vi "Periodic Tasks.vi"(8 "error in":errorcluster) -> ()   [LabVIEW 2020]
doc: "This VI runs in parallel to other tasks. It can contain as many user-defined periodic loops as you need. These can carry out PID or other sorts of timed response."
uses:
  <vilib>/Rock Robotics/WPI/Solenoid/WPI_SolenoidValue.ctl
  <vilib>/Rock Robotics/WPI/ThirdParty/Phoenix-LabVIEW/Motor Controller/Controls/CTRE_Phoenix_MotorControl_ControlMode.ctl
  <vilib>/Rock Robotics/WPI/Utilities/WPI_GetSetVariantRefNum.vi
  Robot Global Data.vi
  <vilib>/Rock Robotics/WPI/Solenoid/WPI_SolenoidSetEnum.vi
  <vilib>/Rock Robotics/Network Tables/NT Write Numeric Array.vi
  <vilib>/Analysis/Matrix/NI_Matrix.lvlib
  <vilib>/Rock Robotics/Network Tables/NT Read Boolean.vi
  <vilib>/Rock Robotics/Network Tables/NT Read String.vi
  <vilib>/Analysis/Matrix/Numeric/Conversions/Matrix To Array - RM.vi
  <vilib>/Utility/file.llb/Write Delimited Spreadsheet (DBL).vi
panel:
  in  "Co Axes Cluster":T1
  in  "Co Button Cluster":T2
  in  "Driver Axes Cluster":T3
  in  "Driver Button Cluster":T4
  out "ArmExtensionEncoderData":i32
  out "ArmPivotEncoderData":i32
  in  "ArmPneumaticControl":T5
  in  "ArmPivotControl":dbl
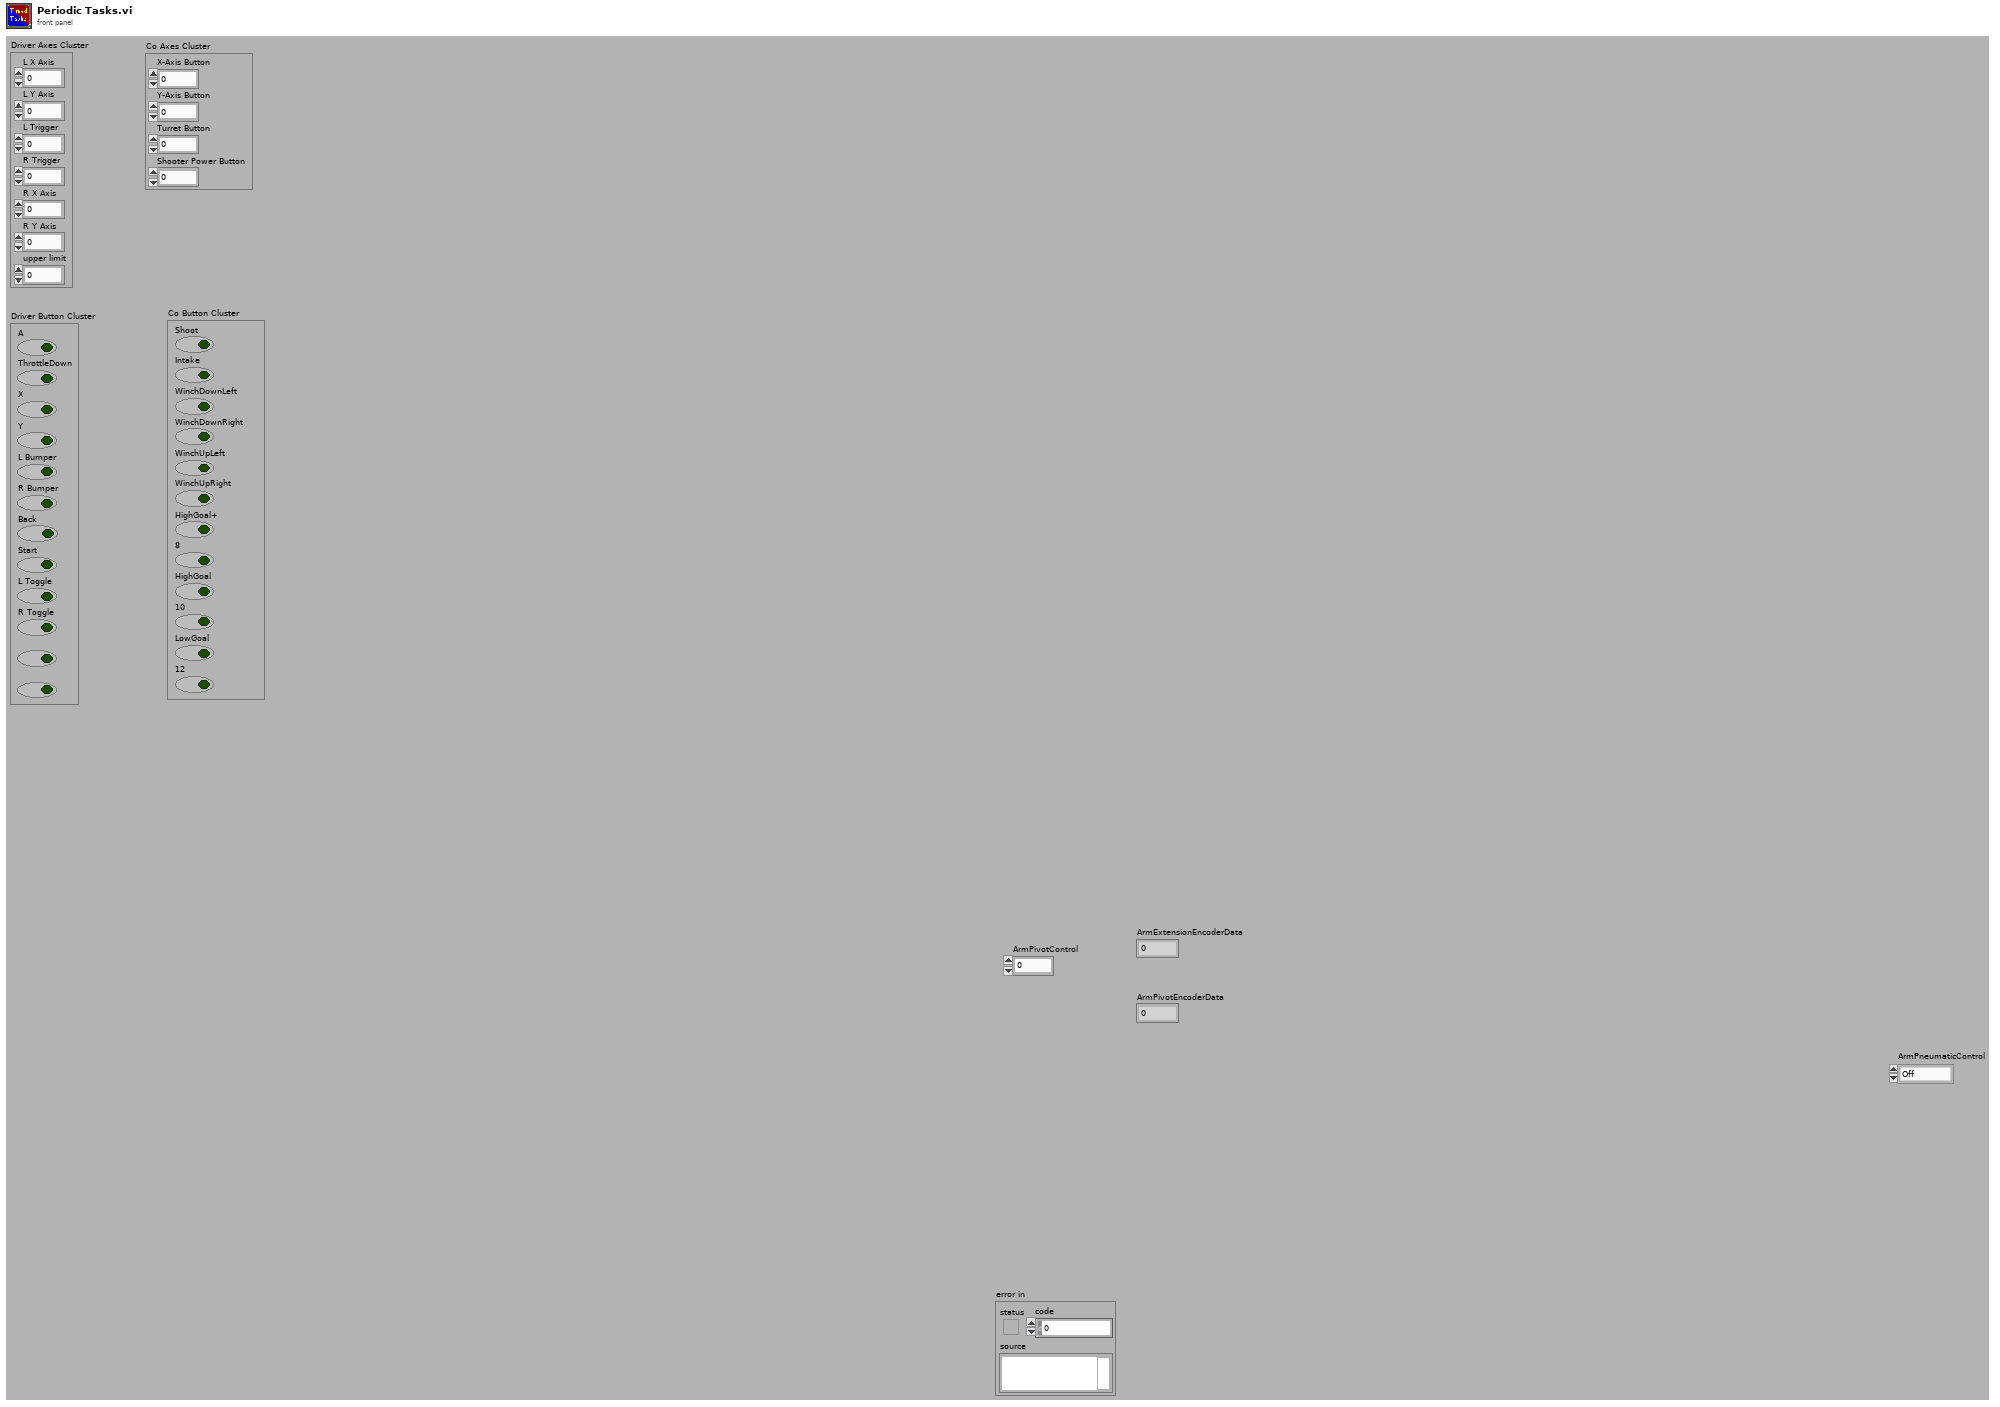
[diagram p1: front panel]
types:
  T1 = cluster{"X-Axis Button":dbl, "Y-Axis Button":dbl, "Turret Button":dbl, "Shooter Power Button":dbl}
  T2 = cluster{"Shoot":bool, "Intake":bool, "WinchDownLeft":bool, "WinchDownRight":bool, "WinchUpLeft":bool, "WinchUpRight":bool, "HighGoal+":bool, "8":bool, "HighGoal":bool, "10":bool, "LowGoal":bool, "12":bool}
  T3 = cluster{"L X Axis":dbl, "L Y Axis":dbl, "L Trigger":dbl, "R Trigger":dbl, "R X Axis":dbl, "R Y Axis":dbl, "upper limit":dbl}
  T4 = cluster{"A":bool, "ThrottleDown":bool, "X":bool, "Y":bool, "L Bumper":bool, "R Bumper":bool, "Back\n":bool, "Start":bool, "L Toggle":bool, "R Toggle":bool, bool, bool}
  T5 = typedef "WPI_SolenoidValue.ctl" = enum16{"Off", "On", "Forward", "Reverse"}
  T6 = typedef "WPI_RobotDriveDevRef.ctl" = cluster{"DevStatus":errorcluster, "Motors[]":T7[], "Square Inputs":bool, "Max Output":dbl}
  T7 = typedef "WPI_MotorControlDeviceRef.ctl" = cluster{"DeviceStatus":errorcluster, "Type":T8, "PWM":cluster{"PWM Channel":T9, "DeadBand":T10}, "CAN":cluster{"Device Number":u8, "SetOutput VI Ref":variant, "GetOutput VI Ref":variant, "Enable VI Ref":variant, "Disable VI Ref":variant, "Data":variant}, "Invert":bool, "DIO PWM":cluster{"PWM \"Enable\" Channel":T9, "DIOChannel":T11, "PWM Rate":dbl}}
  T8 = typedef "WPI_MotorControlType.ctl" = enum16{"PWM", "CAN", "DIO PWM"}
  T9 = typedef "FPGA_DIOPWMChannel.ctl" = enum8{"PWM 0", "PWM 1", "PWM 2", "PWM 3", "PWM 4", "PWM 5", "PWM 6", "PWM 7", "PWM 8", "PWM 9", "PWM MXP 0", "PWM MXP 1", "PWM MXP 2", "PWM MXP 3", "PWM MXP 4", "PWM MXP 5", "PWM MXP 6", "PWM MXP 7", "PWM MXP 8", "PWM MXP 9", "Invalid"}
  T10 = typedef "WPI_PWMDeadband.ctl" = cluster{"Name":string, "maxPositivePwm":i32, "minPositivePwm":i32, "centerPwm":i32, "maxNegativePwm":i32, "minNegativePwm":i32, "angularRange":u16}
  T11 = typedef "FPGA_DIOChannel.ctl" = enum8{"DIO 0", "DIO 1", "DIO 2", "DIO 3", "DIO 4", "DIO 5", "DIO 6", "DIO 7", "DIO 8", "DIO 9", "DIO MXP 0", "DIO MXP 1", "DIO MXP 2", "DIO MXP 3", "DIO MXP 4", "DIO MXP 5", "DIO MXP 6", "DIO MXP 7", "DIO MXP 8", "DIO MXP 9", "DIO MXP 10", "DIO MXP 11", "DIO MXP 12", "DIO MXP 13", "DIO MXP 14", "DIO MXP 15", "SPI Port CS1", "SPI Port CS2", "SPI Port CS3", "SPI Port MISO", "SPI Port MOSI", "Invalid"}
  T12 = typedef "WPI_JoystickDevRef.ctl" = cluster{"Device":T13}
  T13 = typedef "WPI_JoystickDeviceEnum.ctl" = enum16{"USB 0", "USB 1", "USB 2", "USB 3", "USB 4", "USB 5"}
  T14 = typedef "CTRE_Phoenix_MotorControl_ControlMode.ctl" = u16
  T15 = cluster{"JoystickDevRef":T12, "JoystickDevRef":T12, "RobotDriveDevRef":T6}
  T16 = typedef "WPI_DriverStationRobotMode2.ctl" = enum16{"Autonomous Disabled", "Autonomous Enabled", "Teleop Disabled", "Teleop Enabled", "Disconnected", "Finish", "Test Disabled", "Test Enabled", "Emergency Stopped"}
  T17 = typedef "WPI_SolenoidDevRef.ctl" = cluster{"DevStatus":errorcluster, "Pneumatics Control Module":u8, "Forward Solenoid Channel":T18, "Reverse Solenoid Channel":T18}
  T18 = typedef "WPI_SolenoidChannel.ctl" = enum8{"Solenoid 0", "Solenoid 1", "Solenoid 2", "Solenoid 3", "Solenoid 4", "Solenoid 5", "Solenoid 6", "Solenoid 7", "Solenoid 8", "Solenoid 9", "Solenoid 10", "Solenoid 11", "Solenoid 12", "Solenoid 13", "Solenoid 14", "Solenoid 15", "Invalid"}
  T19 = typedef "WPI_DigitalInputDevRef.ctl" = cluster{"DevStatus":errorcluster, "DIO Channel":T11}
  T20 = typedef "WPI_AnalogChannelDevRef.ctl" = cluster{"DevStatus":errorcluster, "Analog Channel":T21}
  T21 = typedef "FPGA_AIChannel.ctl" = enum8{"AI 0", "AI 1", "AI 2", "AI 3", "AI MXP 0", "AI MXP 1", "AI MXP 2", "AI MXP 3", "Invalid"}
  T22 = typedef "CTRE_CANifier_DeviceRef.ctl" = cluster{"DeviceStatus":errorcluster, "Device Number":u8, "Handle":u64, "UsageFrame":u32, "Library Path":path}
  T23 = typedef "NI_Matrix.lvlib/RealMatrix.ctl" = dbl[][]
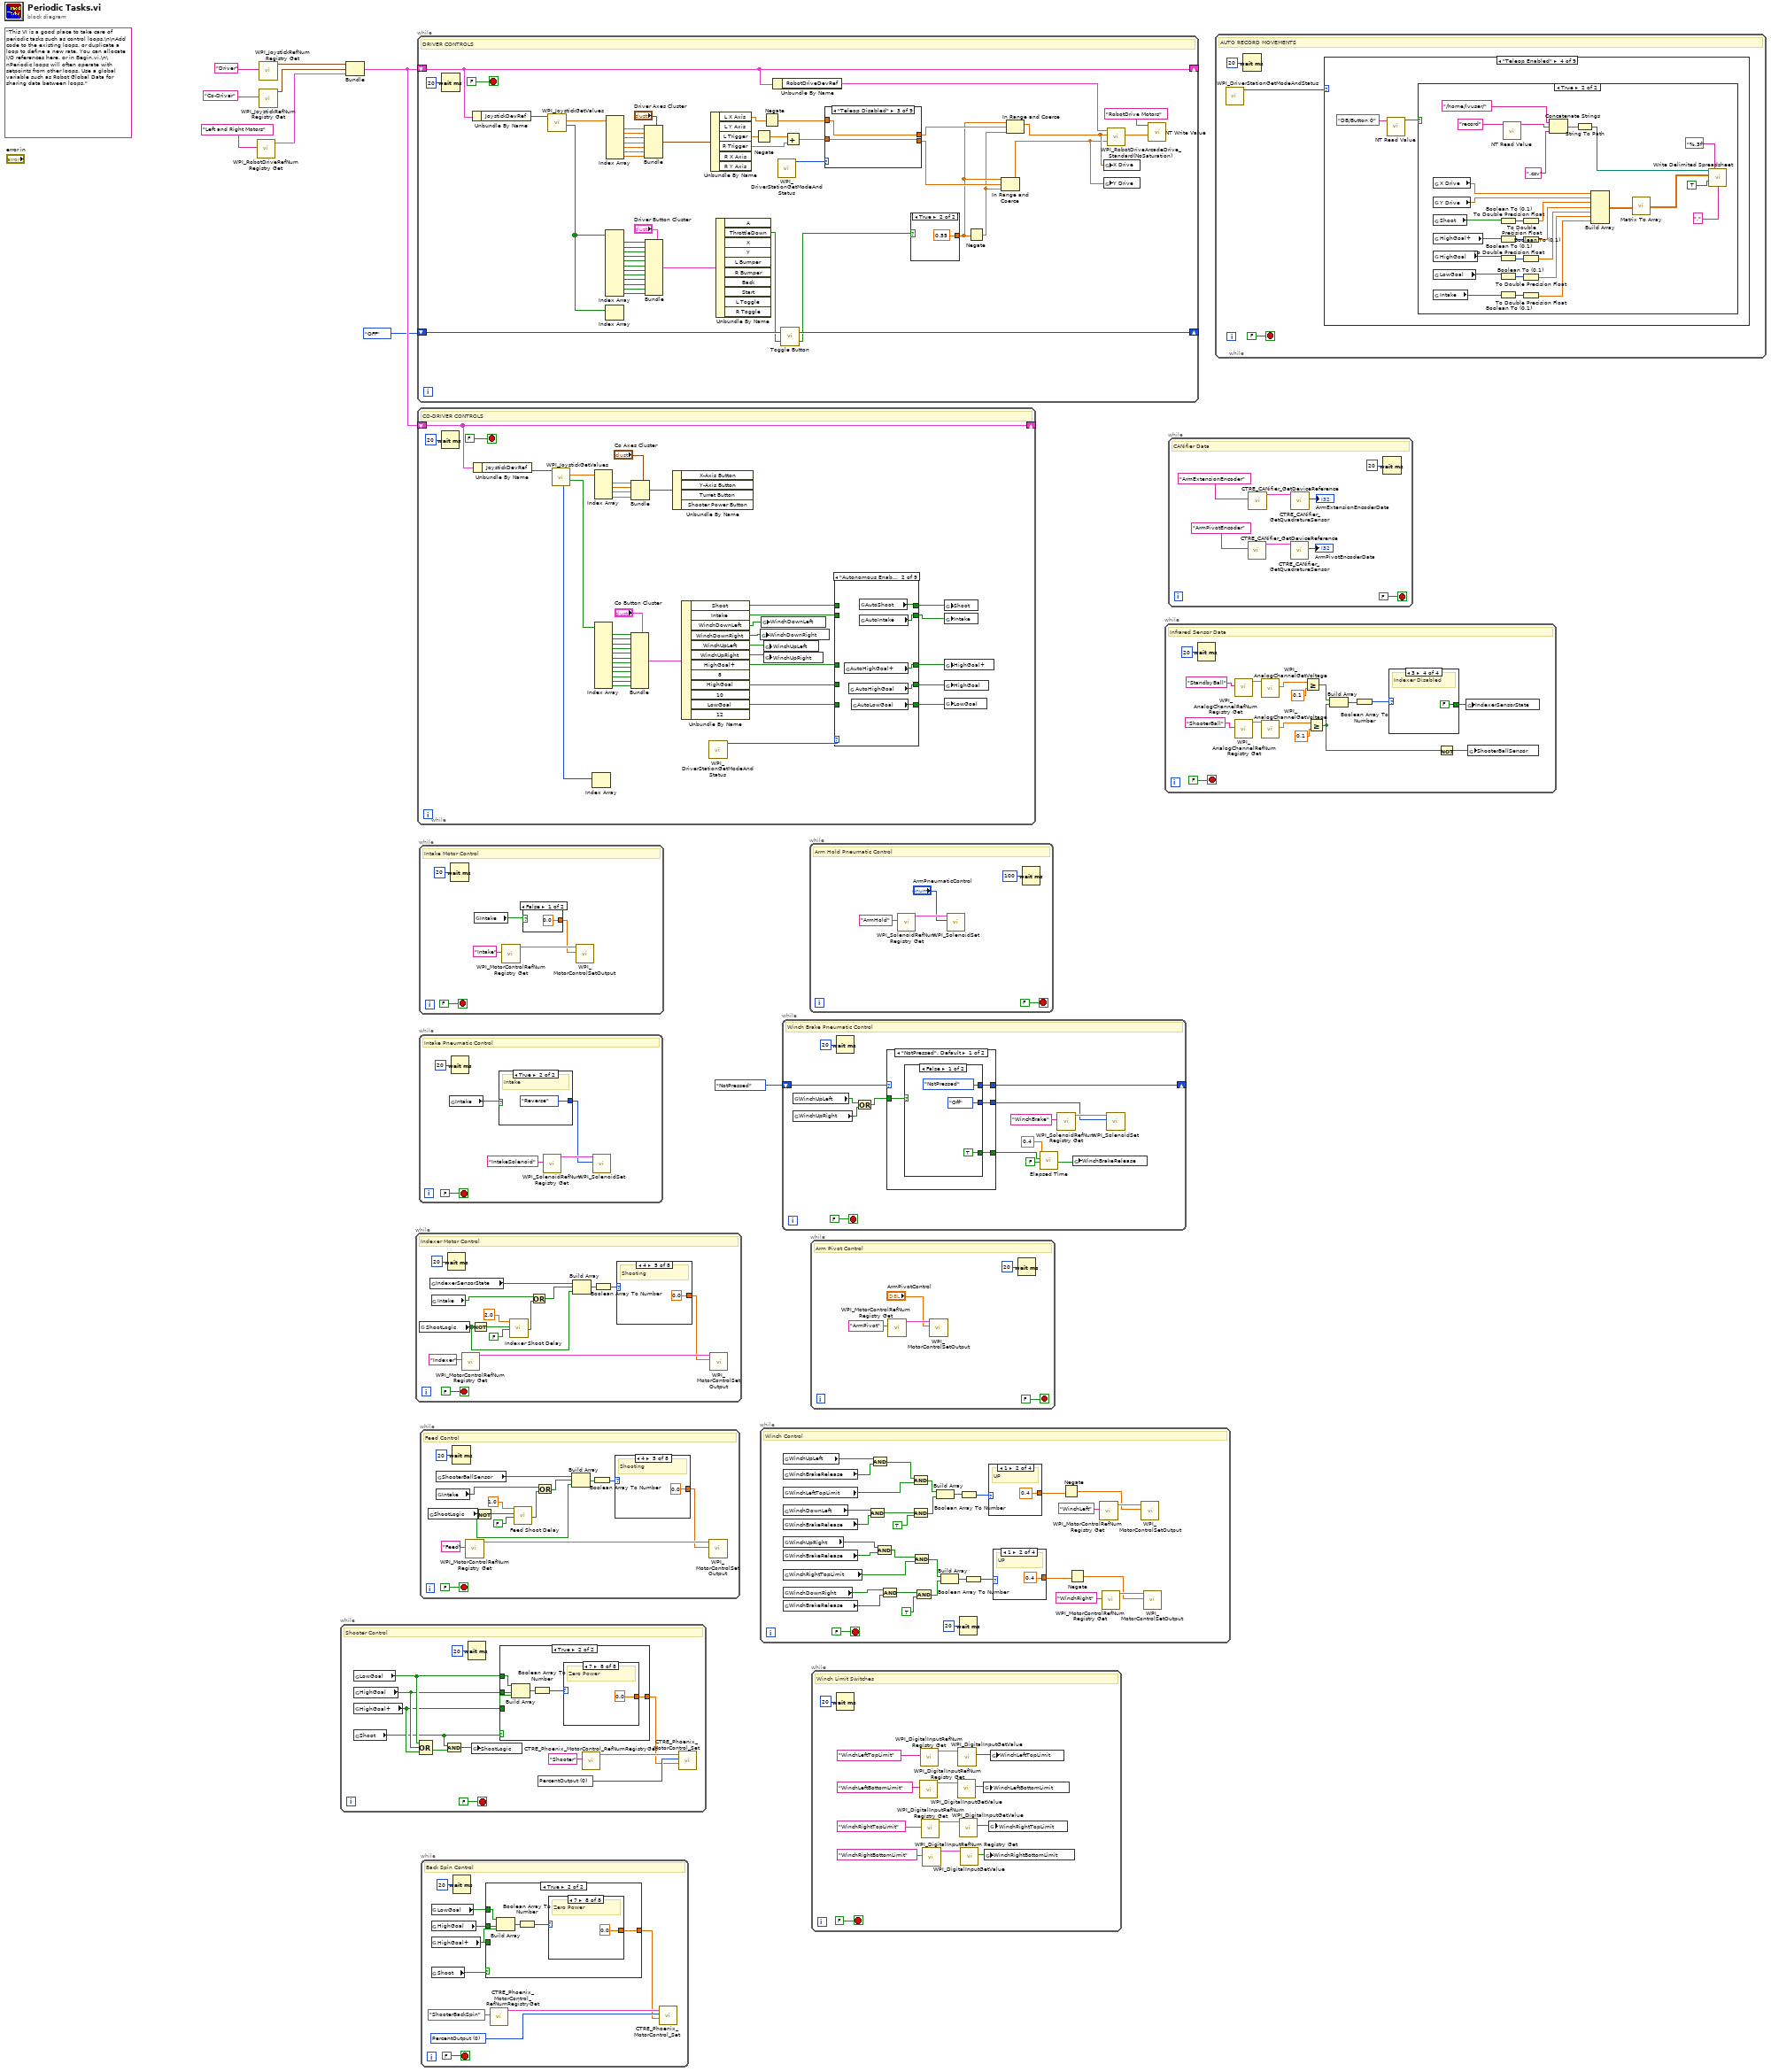
[diagram p0: block diagram]
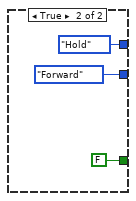
[diagram p11: hidden frame]
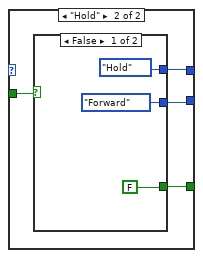
[diagram p12: hidden frame]
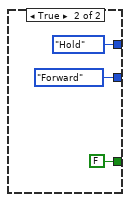
[diagram p13: hidden frame]
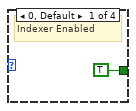
[diagram p14: hidden frame]
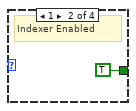
[diagram p15: hidden frame]
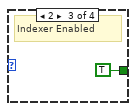
[diagram p16: hidden frame]
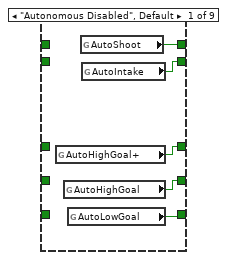
[diagram p17: hidden frame]
diagram:
  (unwired) "This VI is a good place to take care of periodic tasks such as control loops.\n\nAdd code to the existing loops, or duplicate a loop to define a new rate. You can allocate I/O references here, or in Begin.vi.\n\nPeriodic loops will often operate with setpoints from other loops. Use a global variable such as Robot Global Data for sharing data between loops."
  n1 = call <vilib>:"WPI_RobotDriveRefNum Registry Get.vi"("refnum name"="Left and Right Motors") -> ("RobotDriveDevRef"=w6:T6)  [unwired: 1 in, 9 out]
  n2 = call <vilib>:"WPI_JoystickRefNum Registry Get.vi"("refnum name"="Driver") -> ("JoystickDevRef"=w7:T12)  [unwired: 1 in, 9 out]
  n3 = call <vilib>:"WPI_JoystickRefNum Registry Get.vi"("refnum name"="Co-Driver") -> ("JoystickDevRef"=w4:T12)  [unwired: 1 in, 9 out]
  n4 = while {
    stop <- FALSE stop-if-true
    w17 = T14 0 items=["PercentOutput"=0, "Position"=1, "Velocity"=2, "Current"=3, "Follower"=5, "MotionProfile"=6, "MotionMagic"=7, "MotionProfileArc"=10, "Disabled"=15] ("Control Mode")
    # "Shooter Control"
    n5 = global read "Robot Global Data.vi" "LowGoal"() -> (w15:bool)
    n6 = global read "Robot Global Data.vi" "HighGoal"() -> (w14:bool)
    n7 = global read "Robot Global Data.vi" "HighGoal+"() -> (w13:bool)
    n8 = global read "Robot Global Data.vi" "Shoot"() -> (w11:bool)
    n9 = Compound Arithmetic op=OR(w15, w14, w13) -> (w12:bool)
    n10 = And(x=w11, y=w12) -> (x .and. y?=w10:bool)
    n11 = Wait (ms)(milliseconds to wait=u32 20) -> ()  [unwired: 1 out]
    n12 = global write "Robot Global Data.vi" "ShootLogic"(w10) -> ()
    n13 = case shown="True" w11 {
      tunnel: w15 -> [_ w27]
      tunnel: w14 -> [_ w26]
      tunnel: w13 -> [_ w25]
      tunnel: [0.0 w23] -> w16
      frame False {
      }
      frame True {
        n14 = Build Array(w27, w26, w25) -> (w28:bool[])
        n15 = Boolean Array To Number(Boolean array=w28) -> (number=w24:u32)
        n16 = case shown="7" w24 {
          tunnel: [0.0 -0.23 -0.4 0.0 -0.45 0.0 0.0 0.0] -> w23
          frame 0, Default {
            # "Zero Power"
          }
          frame 1 {
            # "Low Goal"
          }
          frame 2 {
            # "High Goal"
          }
          frame 3 {
            # "Zero Power"
          }
          frame 4 {
            # "High Goal +"
          }
          frame 5 {
            # "Zero Power"
          }
          frame 6 {
            # "Zero Power"
          }
          frame 7 {
            # "Zero Power"
          }
        }
      }
    }
    n17 = call <vilib>:"CTRE_Phoenix_MotorControl_RefNumRegistryGet.vi"("refnum name"="Shooter") -> ("PhoenixMotorControlDevRef"=w19:T7)  [unwired: 9 in, 1 out]
    n18 = call <vilib>:"CTRE_Phoenix_MotorControl_Set.vi"("Output"=w16, "Control Mode"=w17, "PhoenixMotorControlDevRef"=w19) -> ()  [unwired: 7 in, 2 out]
  }
  n19 = Bundle("JoystickDevRef"=w7, "JoystickDevRef"=w4, "RobotDriveDevRef"=w6) -> (w3:T15)  [unwired: 1 out]
  n20 = while {
    stop <- FALSE stop-if-true
    # "Indexer Motor Control"
    n21 = global read "Robot Global Data.vi" "ShootLogic"() -> (w38:bool)
    n22 = global read "Robot Global Data.vi" "IndexerSensorState"() -> (w47:bool)
    n23 = global read "Robot Global Data.vi" "Intake"() -> (w40:bool)
    n24 = Wait (ms)(milliseconds to wait=u32 20) -> ()  [unwired: 1 out]
    n25 = call <vilib>:"WPI_MotorControlRefNum Registry Get.vi"("refnum name"="Indexer") -> ("MotorControlDevRef"=w49:T7)  [unwired: 9 in, 1 out]
    n26 = Not(x=w38) -> (.not. x?=w43:bool)
    n27 = call "Indexer Shoot Delay"("Time Target (s)"=2.0, "Reset"=w43, "Auto Reset"=FALSE) -> ("Time has Elapsed"=w37:bool)  [unwired: 9 in, 7 out]
    n28 = Or(x=w40, y=w37) -> (x .or. y?=w39:bool)
    n29 = Build Array(w47, w39, w38) -> (w45:bool[])
    n30 = Boolean Array To Number(Boolean array=w45) -> (number=w46:u32)
    n31 = case shown="4" w46 {
      tunnel: [0.0 0.0 0.0 -0.5 0.0 -1.0 -1.0 -1.0] -> w44
      frame 0, Default {
        # "Zero Power"
      }
      frame 1 {
        # "Zero Power"
      }
      frame 2 {
        # "Zero Power"
      }
      frame 3 {
        # "Intaking"
      }
      frame 4 {
        # "Shooting"
      }
      frame 5 {
        # "Shooting"
      }
      frame 6 {
        # "Shooting"
      }
      frame 7 {
        # "Shooting"
      }
    }
    n32 = call <vilib>:"WPI_MotorControlSetOutput.vi"("Output"=w44, "MotorControlDevRef"=w49) -> ()  [unwired: 7 in, 3 out]
  }
  n33 = while {
    shift-right: [w83] -> _
    shift-left: w3 -> [w83]
    shift-right: [w61] -> _
    shift-left: enum16{"PRESSED ON", "ON", "PRESSED OFF", "OFF"}."OFF" ("State") -> [w63]
    stop <- FALSE stop-if-true
    # "DRIVER CONTROLS"
    n34 = Wait (ms)(milliseconds to wait=u32 20) -> ()  [unwired: 1 out]
    n35 = Unbundle By Name(w83) -> ("JoystickDevRef"=w79:T12)
    n36 = call <vilib>:"WPI_JoystickGetValues.vi"("JoystickDevRef"=w79) -> ("Buttons"=w77:bool[], "Axes"=w78:dbl[])  [unwired: 6 in, 3 out]
    n37 = Index Array(array=w77) -> (element #1=w97:bool, element #2=w96:bool, element #3=w95:bool, element #4=w94:bool, element #5=w93:bool, element #6=w92:bool, element #7=w91:bool, element #8=w90:bool, element #9=w89:bool, element #10=w88:bool, element #11=w87:bool, element #12=w86:bool)  [unwired: 12 in]
    n38 = Index Array(array=w77) -> ()  [unwired: 1 in, 1 out]
    n39 = Index Array(array=w78) -> (element #1=w106:dbl, element #2=w105:dbl, element #3=w104:dbl, element #4=w103:dbl, element #5=w102:dbl, element #6=w101:dbl, element #7=w100:dbl)  [unwired: 7 in]
    n40 = Bundle(cluster="Driver Axes Cluster", "L X Axis"=w106, "L Y Axis"=w105, "L Trigger"=w104, "R Trigger"=w103, "R X Axis"=w102, "R Y Axis"=w101, "upper limit"=w100) -> (w98:T3)
    n41 = Bundle(cluster="Driver Button Cluster", "A"=w97, "ThrottleDown"=w96, "X"=w95, "Y"=w94, "L Bumper"=w93, "R Bumper"=w92, "Back"=w91, "Start"=w90, "L Toggle"=w89, "R Toggle"=w88, w87, w86) -> (w84:T4)
    n42 = Unbundle By Name(w98) -> ("L X Axis"=w73:dbl, "L Trigger"=w76:dbl, "R Trigger"=w74:dbl)  [unwired: 3 out]
    n43 = Unbundle By Name(w84) -> ("ThrottleDown"=w62:bool)  [unwired: 9 out]
    n44 = Negate(x=w76) -> (-x=w75:dbl)
    n45 = Negate(x=w73) -> (-x=w71:dbl)
    n46 = Unbundle By Name(w83) -> ("RobotDriveDevRef"=w82:T6)
    n47 = call <vilib>:"WPI_DriverStationGetModeAndStatus.vi"() -> ("Robot Mode"=w72:T16)  [unwired: 10 in, 1 out]
    n48 = call "Toggle Button.vi"("Button"=w62, "State"=w63) -> ("Output"=w60:bool, "State Output"=w61:enum16{"PRESSED ON", "ON", "PRESSED OFF", "OFF"})
    n49 = Add(x=w75, y=w74) -> (x+y=w70:dbl)
    n50 = case shown="\"Teleop Disabled\"" w72 {
      tunnel: [w112 w114 w116 w118 w120 w122 w124 w126 w128] -> w69
      tunnel: [w111 w113 w115 w117 w119 w121 w123 w125 w127] -> w68
      tunnel: w71 -> [_ _ w116 w118 w120 w122 w124 w126 w128]
      tunnel: w70 -> [_ _ w115 w117 w119 w121 w123 w125 w127]
      frame "Autonomous Disabled", Default {
        n51 = global read "Robot Global Data.vi" "X-DriveAuto"() -> (w112:dbl)
        n52 = global read "Robot Global Data.vi" "Y-DriveAuto"() -> (w111:dbl)
      }
      frame "Autonomous Enabled" {
        n53 = global read "Robot Global Data.vi" "X-DriveAuto"() -> (w114:dbl)
        n54 = global read "Robot Global Data.vi" "Y-DriveAuto"() -> (w113:dbl)
      }
      frame "Teleop Disabled" {
      }
      frame "Teleop Enabled" {
      }
      frame "Disconnected" {
      }
      frame "Finish" {
      }
      frame "Test Disabled" {
      }
      frame "Test Enabled" {
      }
      frame "Emergency Stopped" {
      }
    }
    n55 = case shown="True" w60 {
      tunnel: [0.75 0.55] -> w65
      frame False {
      }
      frame True {
      }
    }
    n56 = Negate(x=w65) -> (-x=w64:dbl)
    n57 = In Range and Coerce(upper limit=w65, x=w68, lower limit=w64) -> (coerced(x)=w66:dbl)  [unwired: 1 out]
    n58 = In Range and Coerce(upper limit=w65, x=w69, lower limit=w64) -> (coerced(x)=w67:dbl)  [unwired: 1 out]
    n59 = global write "Robot Global Data.vi" "X Drive"(w67) -> ()
    n60 = global write "Robot Global Data.vi" "Y Drive"(w66) -> ()
    n61 = call <vilib>:"WPI_RobotDriveArcadeDrive_Standard(NoSaturation).vi"("Y axis value"=w66, "X axis value"=w67, "RobotDriveDevRef"=w82) -> ("Motor Values"=w81:dbl[])  [unwired: 1 in, 7 out]
    n62 = call-poly <vilib>:"NT Write Value.vi"("Numeric Array"=w81, "Name"="RobotDrive Motors") -> ()  [unwired: 9 in, 1 out]
  }
  n63 = while {
    shift-right: [w168] -> _
    shift-left: w3 -> [w168]
    stop <- FALSE stop-if-true
    # "CO-DRIVER CONTROLS"
    n64 = Wait (ms)(milliseconds to wait=u32 20) -> ()  [unwired: 1 out]
    n65 = Unbundle By Name(w168) -> ("JoystickDevRef"=w167:T12)
    n66 = call <vilib>:"WPI_JoystickGetValues.vi"("JoystickDevRef"=w167) -> ("Buttons"=w165:bool[], "Axes"=w166:dbl[], "POVs"=w144:i16[])  [unwired: 6 in, 2 out]
    n67 = Index Array(array=w144) -> ()  [unwired: 1 in, 1 out]
    n68 = Index Array(array=w166) -> (element #1=w164:dbl, element #2=w163:dbl, element #3=w162:dbl, element #4=w161:dbl)  [unwired: 4 in]
    n69 = Index Array(array=w165) -> (element #1=w158:bool, element #2=w157:bool, element #3=w156:bool, element #4=w155:bool, element #5=w154:bool, element #6=w153:bool, element #7=w152:bool, element #8=w151:bool, element #9=w150:bool, element #10=w149:bool, element #11=w148:bool, element #12=w147:bool)  [unwired: 12 in]
    n70 = Bundle(cluster="Co Button Cluster", "Shoot"=w158, "Intake"=w157, "WinchDownLeft"=w156, "WinchDownRight"=w155, "WinchUpLeft"=w154, "WinchUpRight"=w153, "HighGoal+"=w152, "8"=w151, "HighGoal"=w150, "10"=w149, "LowGoal"=w148, "12"=w147) -> (w145:T2)
    n71 = Bundle(cluster="Co Axes Cluster", "X-Axis Button"=w164, "Y-Axis Button"=w163, "Turret Button"=w162, "Shooter Power Button"=w161) -> (w159:T1)
    n72 = Unbundle By Name(w159) -> ()  [unwired: 4 out]
    n73 = Unbundle By Name(w145) -> ("Shoot"=w142:bool, "Intake"=w140:bool, "WinchDownLeft"=w130:bool, "WinchDownRight"=w131:bool, "WinchUpLeft"=w129:bool, "WinchUpRight"=w132:bool, "HighGoal+"=w138:bool, "HighGoal"=w136:bool, "LowGoal"=w134:bool)  [unwired: 3 out]
    n74 = call <vilib>:"WPI_DriverStationGetModeAndStatus.vi"() -> ("Robot Mode"=w143:T16)  [unwired: 10 in, 1 out]
    n75 = global write "Robot Global Data.vi" "WinchDownRight"(w131) -> ()
    n76 = global write "Robot Global Data.vi" "WinchDownLeft"(w130) -> ()
    n77 = global write "Robot Global Data.vi" "WinchUpLeft"(w129) -> ()
    n78 = global write "Robot Global Data.vi" "WinchUpRight"(w132) -> ()
    n79 = case shown="\"Autonomous Enabled\"" w143 {
      tunnel: [w175 w180 w185 w190 w195 w200 w205 w210 w215] -> w141
      tunnel: w142 -> [_ _ w185 w190 w195 w200 w205 w210 w215]
      tunnel: [w174 w179 w184 w189 w194 w199 w204 w209 w214] -> w139
      tunnel: w140 -> [_ _ w184 w189 w194 w199 w204 w209 w214]
      tunnel: [w173 w178 w183 w188 w193 w198 w203 w208 w213] -> w137
      tunnel: w138 -> [_ _ w183 w188 w193 w198 w203 w208 w213]
      tunnel: [w172 w177 w182 w187 w192 w197 w202 w207 w212] -> w135
      tunnel: w136 -> [_ _ w182 w187 w192 w197 w202 w207 w212]
      tunnel: [w171 w176 w181 w186 w191 w196 w201 w206 w211] -> w133
      tunnel: w134 -> [_ _ w181 w186 w191 w196 w201 w206 w211]
      frame "Autonomous Disabled", Default {
        n80 = global read "Robot Global Data.vi" "AutoHighGoal+"() -> (w173:bool)
        n81 = global read "Robot Global Data.vi" "AutoHighGoal"() -> (w172:bool)
        n82 = global read "Robot Global Data.vi" "AutoLowGoal"() -> (w171:bool)
        n83 = global read "Robot Global Data.vi" "AutoShoot"() -> (w175:bool)
        n84 = global read "Robot Global Data.vi" "AutoIntake"() -> (w174:bool)
      }
      frame "Autonomous Enabled" {
        n85 = global read "Robot Global Data.vi" "AutoHighGoal+"() -> (w178:bool)
        n86 = global read "Robot Global Data.vi" "AutoHighGoal"() -> (w177:bool)
        n87 = global read "Robot Global Data.vi" "AutoLowGoal"() -> (w176:bool)
        n88 = global read "Robot Global Data.vi" "AutoShoot"() -> (w180:bool)
        n89 = global read "Robot Global Data.vi" "AutoIntake"() -> (w179:bool)
      }
      frame "Teleop Disabled" {
      }
      frame "Teleop Enabled" {
      }
      frame "Disconnected" {
      }
      frame "Finish" {
      }
      frame "Test Disabled" {
      }
      frame "Test Enabled" {
      }
      frame "Emergency Stopped" {
      }
    }
    n90 = global write "Robot Global Data.vi" "Shoot"(w141) -> ()
    n91 = global write "Robot Global Data.vi" "Intake"(w139) -> ()
    n92 = global write "Robot Global Data.vi" "HighGoal+"(w137) -> ()
    n93 = global write "Robot Global Data.vi" "HighGoal"(w135) -> ()
    n94 = global write "Robot Global Data.vi" "LowGoal"(w133) -> ()
  }
  n95 = while {
    stop <- FALSE stop-if-true
    # "Intake Pneumatic Control"
    n96 = global read "Robot Global Data.vi" "Intake"() -> (w217:bool)
    n97 = Wait (ms)(milliseconds to wait=u32 20) -> ()  [unwired: 1 out]
    n98 = case shown="True" w217 {
      tunnel: [WPI_SolenoidValue."Forward" ("IntakePneumaticControl") WPI_SolenoidValue."Reverse" ("IntakePneumaticControl")] -> w216
      frame False {
        # "Retract"
      }
      frame True {
        # "Intake"
      }
    }
    n99 = call <vilib>:"WPI_SolenoidRefNum Registry Get.vi"("refnum name"="IntakeSolenoid") -> ("SolenoidDevRef"=w219:T17)  [unwired: 9 in, 1 out]
    n100 = call-poly <vilib>:"WPI_SolenoidSet.vi"("Value"=w216, "SolenoidDevRef"=w219) -> ()  [unwired: 8 in, 2 out]
  }
  n101 = while {
    stop <- FALSE stop-if-true
    # "Intake Motor Control"
    n102 = Wait (ms)(milliseconds to wait=u32 20) -> ()  [unwired: 1 out]
    n103 = global read "Robot Global Data.vi" "Intake"() -> (w225:bool)
    n104 = call <vilib>:"WPI_MotorControlRefNum Registry Get.vi"("refnum name"="Intake") -> ("MotorControlDevRef"=w227:T7)  [unwired: 9 in, 1 out]
    n105 = case shown="False" w225 {
      tunnel: [0.0 1.0] -> w224
      frame False {
      }
      frame True {
      }
    }
    n106 = call <vilib>:"WPI_MotorControlSetOutput.vi"("Output"=w224, "MotorControlDevRef"=w227) -> ()  [unwired: 7 in, 3 out]
  }
  n107 = while {
    stop <- FALSE stop-if-true
    # "Feed Control"
    n108 = global read "Robot Global Data.vi" "ShootLogic"() -> (w233:bool)
    n109 = global read "Robot Global Data.vi" "ShooterBallSensor"() -> (w242:bool)
    n110 = global read "Robot Global Data.vi" "Intake"() -> (w235:bool)
    n111 = Wait (ms)(milliseconds to wait=u32 20) -> ()  [unwired: 1 out]
    n112 = call <vilib>:"WPI_MotorControlRefNum Registry Get.vi"("refnum name"="Feed") -> ("MotorControlDevRef"=w244:T7)  [unwired: 9 in, 1 out]
    n113 = Not(x=w233) -> (.not. x?=w238:bool)
    n114 = call "Feed Shoot Delay"("Time Target (s)"=1.0, "Reset"=w238, "Auto Reset"=FALSE) -> ("Time has Elapsed"=w232:bool)  [unwired: 9 in, 7 out]
    n115 = Or(x=w235, y=w232) -> (x .or. y?=w234:bool)
    n116 = Build Array(w242, w234, w233) -> (w240:bool[])
    n117 = Boolean Array To Number(Boolean array=w240) -> (number=w241:u32)
    n118 = case shown="4" w241 {
      tunnel: [0.0 0.0 0.0 0.25 0.0 1.0 1.0 1.0] -> w239
      frame 0, Default {
        # "Zero Power"
      }
      frame 1 {
        # "Zero Power"
      }
      frame 2 {
        # "Zero Power"
      }
      frame 3 {
        # "Intaking"
      }
      frame 4 {
        # "Shooting"
      }
      frame 5 {
        # "Shooting"
      }
      frame 6 {
        # "Shooting"
      }
      frame 7 {
        # "Shooting"
      }
    }
    n119 = call <vilib>:"WPI_MotorControlSetOutput.vi"("Output"=w239, "MotorControlDevRef"=w244) -> ()  [unwired: 7 in, 3 out]
  }
  n120 = while {
    stop <- FALSE stop-if-true
    w261 = T14 0 items=["PercentOutput"=0, "Position"=1, "Velocity"=2, "Current"=3, "Follower"=5, "MotionProfile"=6, "MotionMagic"=7, "MotionProfileArc"=10, "Disabled"=15] ("Control Mode")
    # "Back Spin Control"
    n121 = global read "Robot Global Data.vi" "LowGoal"() -> (w259:bool)
    n122 = global read "Robot Global Data.vi" "HighGoal"() -> (w258:bool)
    n123 = global read "Robot Global Data.vi" "HighGoal+"() -> (w257:bool)
    n124 = global read "Robot Global Data.vi" "Shoot"() -> (w255:bool)
    n125 = Wait (ms)(milliseconds to wait=u32 20) -> ()  [unwired: 1 out]
    n126 = case shown="True" w255 {
      tunnel: w259 -> [_ w270]
      tunnel: w258 -> [_ w269]
      tunnel: w257 -> [_ w268]
      tunnel: [0.0 w266] -> w256
      frame False {
      }
      frame True {
        n127 = Build Array(w270, w269, w268) -> (w271:bool[])
        n128 = Boolean Array To Number(Boolean array=w271) -> (number=w267:u32)
        n129 = case shown="7" w267 {
          tunnel: [0.0 -0.23 -0.4 0.0 -0.45 0.0 0.0 0.0] -> w266
          frame 0, Default {
            # "Zero Power"
          }
          frame 1 {
            # "Low Goal"
          }
          frame 2 {
            # "High Goal"
          }
          frame 3 {
            # "Zero Power"
          }
          frame 4 {
            # "High Goal +"
          }
          frame 5 {
            # "Zero Power"
          }
          frame 6 {
            # "Zero Power"
          }
          frame 7 {
            # "Zero Power"
          }
        }
      }
    }
    n130 = call <vilib>:"CTRE_Phoenix_MotorControl_RefNumRegistryGet.vi"("refnum name"="ShooterBackSpin") -> ("PhoenixMotorControlDevRef"=w262:T7)  [unwired: 9 in, 1 out]
    n131 = call <vilib>:"CTRE_Phoenix_MotorControl_Set.vi"("Output"=w256, "Control Mode"=w261, "PhoenixMotorControlDevRef"=w262) -> ()  [unwired: 7 in, 2 out]
  }
  n132 = while {
    stop <- FALSE stop-if-true
    # "Winch Control"
    n133 = global read "Robot Global Data.vi" "WinchUpLeft"() -> (w285:bool)
    n134 = global read "Robot Global Data.vi" "WinchBrakeRelease"() -> (w284:bool)
    n135 = global read "Robot Global Data.vi" "WinchLeftTopLimit"() -> (w307:bool)
    n136 = global read "Robot Global Data.vi" "WinchDownLeft"() -> (w282:bool)
    n137 = global read "Robot Global Data.vi" "WinchBrakeRelease"() -> (w281:bool)
    n138 = global read "Robot Global Data.vi" "WinchUpRight"() -> (w291:bool)
    n139 = global read "Robot Global Data.vi" "WinchBrakeRelease"() -> (w290:bool)
    n140 = global read "Robot Global Data.vi" "WinchRightTopLimit"() -> (w306:bool)
    n141 = global read "Robot Global Data.vi" "WinchDownRight"() -> (w288:bool)
    n142 = global read "Robot Global Data.vi" "WinchBrakeRelease"() -> (w286:bool)
    n143 = And(x=w282, y=w281) -> (x .and. y?=w280:bool)
    n144 = And(x=w285, y=w284) -> (x .and. y?=w283:bool)
    n145 = And(x=w291, y=w290) -> (x .and. y?=w289:bool)
    n146 = And(x=w288, y=w286) -> (x .and. y?=w287:bool)
    n147 = And(x=w283, y=w307) -> (x .and. y?=w305:bool)
    n148 = And(x=w280, y=TRUE) -> (x .and. y?=w304:bool)
    n149 = And(x=w289, y=w306) -> (x .and. y?=w299:bool)
    n150 = And(x=w287, y=TRUE) -> (x .and. y?=w298:bool)
    n151 = Build Array(w305, w304) -> (w303:bool[])
    n152 = Build Array(w299, w298) -> (w301:bool[])
    n153 = Wait (ms)(milliseconds to wait=u32 20) -> ()  [unwired: 1 out]
    n154 = Boolean Array To Number(Boolean array=w303) -> (number=w302:u32)
    n155 = Boolean Array To Number(Boolean array=w301) -> (number=w300:u32)
    n156 = case shown="1" w302 {
      tunnel: [0.0 0.4 -1.0 0.0] -> w297
      frame 0, Default {
        # "STOP"
      }
      frame 1 {
        # "UP"
      }
      frame 2 {
        # "DOWN"
      }
      frame 3 {
        # "STOP"
      }
    }
    n157 = case shown="1" w300 {
      tunnel: [0.0 0.4 -1.0 0.0] -> w295
      frame 0, Default {
        # "STOP"
      }
      frame 1 {
        # "UP"
      }
      frame 2 {
        # "DOWN"
      }
      frame 3 {
        # "STOP"
      }
    }
    n158 = Negate(x=w297) -> (-x=w296:dbl)
    n159 = Negate(x=w295) -> (-x=w294:dbl)
    n160 = call <vilib>:"WPI_MotorControlRefNum Registry Get.vi"("refnum name"="WinchLeft") -> ("MotorControlDevRef"=w311:T7)  [unwired: 9 in, 1 out]
    n161 = call <vilib>:"WPI_MotorControlRefNum Registry Get.vi"("refnum name"="WinchRight") -> ("MotorControlDevRef"=w308:T7)  [unwired: 9 in, 1 out]
    n162 = call <vilib>:"WPI_MotorControlSetOutput.vi"("Output"=w296, "MotorControlDevRef"=w311) -> ()  [unwired: 7 in, 3 out]
    n163 = call <vilib>:"WPI_MotorControlSetOutput.vi"("Output"=w294, "MotorControlDevRef"=w308) -> ()  [unwired: 7 in, 3 out]
  }
  n164 = while {
    shift-right: [w330] -> _
    shift-left: enum16{"NotPressed", "Hold"}."NotPressed" -> [w331]
    stop <- FALSE stop-if-true
    # "Winch Brake Pneumatic Control"
    n165 = global read "Robot Global Data.vi" "WinchUpRight"() -> (w323:bool)
    n166 = global read "Robot Global Data.vi" "WinchUpLeft"() -> (w324:bool)
    n167 = Wait (ms)(milliseconds to wait=u32 20) -> ()  [unwired: 1 out]
    n168 = Or(x=w324, y=w323) -> (x .or. y?=w322:bool)
    n169 = case shown="\"NotPressed\", Default" w331 {
      tunnel: w322 -> [w339 w348]
      tunnel: [w338 w349] -> w330
      tunnel: [w337 w347] -> w329
      tunnel: [w336 w346] -> w325
      frame "NotPressed", Default {
        n170 = case shown="False" w339 {
          tunnel: [enum16{"NotPressed", "Hold"}."NotPressed" enum16{"NotPressed", "Hold"}."Hold"] -> w338
          tunnel: [WPI_SolenoidValue."Off" ("Value") WPI_SolenoidValue."Forward" ("Value")] -> w337
          tunnel: [TRUE ("Auto Reset") FALSE ("Auto Reset")] -> w336
          frame False {
          }
          frame True {
          }
        }
      }
      frame "Hold" {
        n171 = case shown="False" w348 {
          tunnel: [enum16{"NotPressed", "Hold"}."Hold" enum16{"NotPressed", "Hold"}."Hold"] -> w349
          tunnel: [WPI_SolenoidValue."Forward" ("Value") WPI_SolenoidValue."Forward" ("Value")] -> w347
          tunnel: [FALSE ("Auto Reset") FALSE ("Auto Reset")] -> w346
          frame False {
          }
          frame True {
          }
        }
      }
    }
    n172 = call "Elapsed Time"("Time Target (s)"=0.4, "Reset"=w325, "Auto Reset"=FALSE) -> ("Time has Elapsed"=w326:bool)  [unwired: 9 in, 7 out]
    n173 = call <vilib>:"WPI_SolenoidRefNum Registry Get.vi"("refnum name"="WinchBrake") -> ("SolenoidDevRef"=w333:T17)  [unwired: 9 in, 1 out]
    n174 = global write "Robot Global Data.vi" "WinchBrakeRelease"(w326) -> ()
    n175 = call-poly <vilib>:"WPI_SolenoidSet.vi"("Value"=w329, "SolenoidDevRef"=w333) -> ()  [unwired: 8 in, 2 out]
  }
  n176 = while {
    stop <- FALSE stop-if-true
    # "Arm Hold Pneumatic Control"
    n177 = call <vilib>:"WPI_SolenoidRefNum Registry Get.vi"("refnum name"="ArmHold") -> ("SolenoidDevRef"=w358:T17)  [unwired: 9 in, 1 out]
    n178 = call-poly <vilib>:"WPI_SolenoidSet.vi"("Value"="ArmPneumaticControl", "SolenoidDevRef"=w358) -> ()  [unwired: 8 in, 2 out]
    n179 = Wait (ms)(milliseconds to wait=u32 100) -> ()  [unwired: 1 out]
  }
  n180 = while {
    stop <- FALSE stop-if-true
    # "Arm Pivot Control"
    n181 = call <vilib>:"WPI_MotorControlRefNum Registry Get.vi"("refnum name"="ArmPivot") -> ("MotorControlDevRef"=w363:T7)  [unwired: 9 in, 1 out]
    n182 = call <vilib>:"WPI_MotorControlSetOutput.vi"("Output"="ArmPivotControl", "MotorControlDevRef"=w363) -> ()  [unwired: 7 in, 3 out]
    n183 = Wait (ms)(milliseconds to wait=u32 20) -> ()  [unwired: 1 out]
  }
  n184 = while {
    stop <- FALSE stop-if-true
    # "Winch Limit Switches"
    n185 = Wait (ms)(milliseconds to wait=u32 20) -> ()  [unwired: 1 out]
    n186 = call <vilib>:"WPI_DigitalInputRefNum Registry Get.vi"("refnum name"="WinchLeftBottomLimit") -> ("DigitalInputDevRef"=w373:T19)  [unwired: 9 in, 1 out]
    n187 = call <vilib>:"WPI_DigitalInputRefNum Registry Get.vi"("refnum name"="WinchLeftTopLimit") -> ("DigitalInputDevRef"=w376:T19)  [unwired: 9 in, 1 out]
    n188 = call <vilib>:"WPI_DigitalInputRefNum Registry Get.vi"("refnum name"="WinchRightTopLimit") -> ("DigitalInputDevRef"=w370:T19)  [unwired: 9 in, 1 out]
    n189 = call <vilib>:"WPI_DigitalInputRefNum Registry Get.vi"("refnum name"="WinchRightBottomLimit") -> ("DigitalInputDevRef"=w367:T19)  [unwired: 9 in, 1 out]
    n190 = call <vilib>:"WPI_DigitalInputGetValue.vi"("DigitalInputDevRef"=w373) -> ("Value"=w372:bool)  [unwired: 8 in, 2 out]
    n191 = call <vilib>:"WPI_DigitalInputGetValue.vi"("DigitalInputDevRef"=w376) -> ("Value"=w375:bool)  [unwired: 8 in, 2 out]
    n192 = call <vilib>:"WPI_DigitalInputGetValue.vi"("DigitalInputDevRef"=w370) -> ("Value"=w369:bool)  [unwired: 8 in, 2 out]
    n193 = call <vilib>:"WPI_DigitalInputGetValue.vi"("DigitalInputDevRef"=w367) -> ("Value"=w366:bool)  [unwired: 8 in, 2 out]
    n194 = global write "Robot Global Data.vi" "WinchLeftBottomLimit"(w372) -> ()
    n195 = global write "Robot Global Data.vi" "WinchRightBottomLimit"(w366) -> ()
    n196 = global write "Robot Global Data.vi" "WinchRightTopLimit"(w369) -> ()
    n197 = global write "Robot Global Data.vi" "WinchLeftTopLimit"(w375) -> ()
  }
  n198 = while {
    stop <- FALSE stop-if-true
    # "Infrared Sensor Data"
    n199 = Wait (ms)(milliseconds to wait=u32 20) -> ()  [unwired: 1 out]
    n200 = call <vilib>:"WPI_AnalogChannelRefNum Registry Get.vi"("refnum name"="StandbyBall") -> ("AIDeviceRef"=w384:T20)  [unwired: 9 in, 1 out]
    n201 = call <vilib>:"WPI_AnalogChannelRefNum Registry Get.vi"("refnum name"="ShooterBall") -> ("AIDeviceRef"=w382:T20)  [unwired: 9 in, 1 out]
    n202 = call <vilib>:"WPI_AnalogChannelGetVoltage.vi"("AIDeviceRef"=w384) -> ("Voltage"=w383:dbl)  [unwired: 8 in, 2 out]
    n203 = call <vilib>:"WPI_AnalogChannelGetVoltage.vi"("AIDeviceRef"=w382) -> ("Voltage"=w380:dbl)  [unwired: 8 in, 2 out]
    n204 = Greater Or Equal?(x=w383, y=0.1) -> (x >= y?=w391:bool)
    n205 = Greater Or Equal?(x=w380, y=0.1) -> (x >= y?=w386:bool)
    n206 = Build Array(w391, w386) -> (w390:bool[])
    n207 = Boolean Array To Number(Boolean array=w390) -> (number=w389:u32)
    n208 = case shown="3" w389 {
      tunnel: [TRUE TRUE TRUE FALSE] -> w388
      frame 0, Default {
        # "Indexer Enabled"
      }
      frame 1 {
        # "Indexer Enabled"
      }
      frame 2 {
        # "Indexer Enabled"
      }
      frame 3 {
        # "Indexer Disabled"
      }
    }
    n209 = Not(x=w386) -> (.not. x?=w387:bool)
    n210 = global write "Robot Global Data.vi" "IndexerSensorState"(w388) -> ()
    n211 = global write "Robot Global Data.vi" "ShooterBallSensor"(w387) -> ()
  }
  n212 = while {
    stop <- FALSE stop-if-true
    # "CANifier Data"
    n213 = call <vilib>:"CTRE_CANifier_GetDeviceReference.vi"("refnum name"="ArmPivotEncoder") -> ("CANifierDevRef"=w403:T22)  [unwired: 9 in, 1 out]
    n214 = call <vilib>:"CTRE_CANifier_GetDeviceReference.vi"("refnum name"="ArmExtensionEncoder") -> ("CANifierDevRef"=w406:T22)  [unwired: 9 in, 1 out]
    n215 = call <vilib>:"CTRE_CANifier_GetQuadratureSensor.vi"("CANifierDevRef"=w403) -> ("pos"=→"ArmPivotEncoderData":i32)  [unwired: 7 in, 3 out]
    n216 = call <vilib>:"CTRE_CANifier_GetQuadratureSensor.vi"("CANifierDevRef"=w406) -> ("pos"=→"ArmExtensionEncoderData":i32)  [unwired: 7 in, 3 out]
    n217 = Wait (ms)(milliseconds to wait=u32 20) -> ()  [unwired: 1 out]
  }
  n218 = while {
    stop <- FALSE stop-if-true
    # "AUTO RECORD MOVEMENTS"
    n219 = call <vilib>:"WPI_DriverStationGetModeAndStatus.vi"() -> ("Robot Mode"=w408:T16)  [unwired: 10 in, 1 out]
    n220 = Wait (ms)(milliseconds to wait=u32 20) -> ()  [unwired: 1 out]
    n221 = case shown="\"Teleop Enabled\"" w408 {
      frame "Autonomous Disabled", Default {
      }
      frame "Autonomous Enabled" {
      }
      frame "Teleop Disabled" {
      }
      frame "Teleop Enabled" {
        n222 = call-poly <vilib>:"NT Read Value.vi"("Name"="DB/Button 0" ("refnum name")) -> ("Boolean"=w411:bool)  [unwired: 9 in, 1 out]
        n223 = case shown="True" w411 {
          frame False {
          }
          frame True {
            n224 = global read "Robot Global Data.vi" "X Drive"() -> (w414:dbl)
            n225 = global read "Robot Global Data.vi" "Y Drive"() -> (w413:dbl)
            n226 = global read "Robot Global Data.vi" "Shoot"() -> (w438:bool)
            n227 = global read "Robot Global Data.vi" "HighGoal+"() -> (w437:bool)
            n228 = global read "Robot Global Data.vi" "HighGoal"() -> (w436:bool)
            n229 = global read "Robot Global Data.vi" "LowGoal"() -> (w435:bool)
            n230 = global read "Robot Global Data.vi" "Intake"() -> (w434:bool)
            n231 = Boolean To (0,1)(Boolean=w438) -> (0, 1=w433:i16)
            n232 = Boolean To (0,1)(Boolean=w437) -> (0, 1=w432:i16)
            n233 = Boolean To (0,1)(Boolean=w436) -> (0, 1=w431:i16)
            n234 = Boolean To (0,1)(Boolean=w435) -> (0, 1=w430:i16)
            n235 = Boolean To (0,1)(Boolean=w434) -> (0, 1=w429:i16)
            n236 = call-poly <vilib>:"NT Read Value.vi"("Name"="record") -> ("String"=w418:string)  [unwired: 9 in, 1 out]
            n237 = To Double Precision Float(number=w433) -> (double precision float=w428:dbl)
            n238 = To Double Precision Float(number=w432) -> (double precision float=w427:dbl)
            n239 = To Double Precision Float(number=w431) -> (double precision float=w426:dbl)
            n240 = To Double Precision Float(number=w430) -> (double precision float=w425:dbl)
            n241 = To Double Precision Float(number=w429) -> (double precision float=w424:dbl)
            n242 = Concatenate Strings("/home/lvuser/", w418, ".csv") -> (w416:string)
            n243 = String To Path(string=w416) -> (path=w415:path)
            n244 = Build Array(w414, w413, w428, w427, w426, w425, w424) -> (w440:T23)
            n245 = call-poly <vilib>:"Matrix To Array.vi"("Real Matrix"=w440) -> ("Real 2D Array"=w439:dbl[][])
            n246 = call-poly <vilib>:"Write Delimited Spreadsheet.vi"("file path (dialog if empty)"=w415, "format (%.3f)"="%.3f", "2D data"=w439, "append to file? (new file:F)"=TRUE, "delimiter (\\t)"="," ("delimiter (\\t)")) -> ()  [unwired: 9 in, 2 out]
          }
        }
      }
      frame "Disconnected" {
      }
      frame "Finish" {
      }
      frame "Test Disabled" {
      }
      frame "Test Enabled" {
      }
      frame "Emergency Stopped" {
      }
    }
  }
